vi "transition.vi"(8 "error in (no error)":errorcluster, 10 "Context In":refnum<class "Context.lvclass">, 11 "Exit in":refnum<class "Exit.lvclass">) -> (0 "error out":errorcluster, 2 "Context Out":refnum<class "Context.lvclass">, 3 "Exit out":refnum<class "Exit.lvclass">)   [LabVIEW 2018, in "Exit.lvclass"]
uses:
  Exit.lvclass
  C:/Users/fflores/Documents/OOP-State-Machine/State/State.lvclass
  Context/Context.lvclass
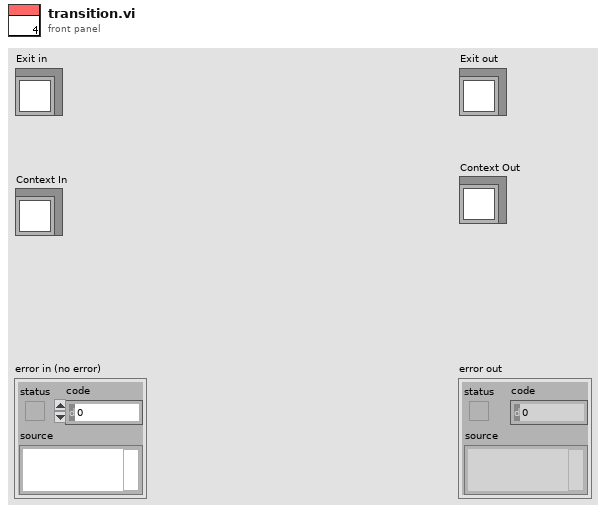
[diagram p1: front panel]
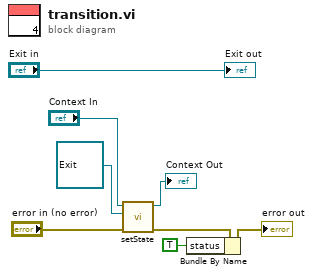
[diagram p0: block diagram]
diagram:
  n1 = call "setState.vi"("error in (no error)"="error in (no error)", "State.lvclass"=refnum<class "Exit.lvclass"> refnum ("Run.lvclass"), "Context in"="Context In") -> ("error out"=w6:errorcluster, "Context out"=→"Context Out":refnum<class "Context.lvclass">)  [unwired: 7 in]
  n2 = Bundle By Name(cluster=w6, "status"=TRUE) -> (→"error out":errorcluster)
  "Exit out" <- "Exit in"
